vi "Get-Power.vi"(8 "error in":errorcluster, 11 "Average Time (0.0)":dbl=0.1) -> (0 "error out":errorcluster, 3 "Power":dbl)   [LabVIEW 2014]
uses:
  Global variables.vi
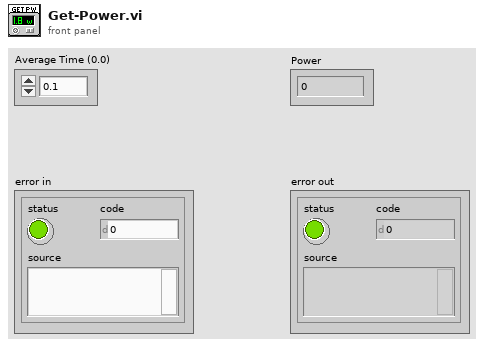
[diagram p1: front panel]
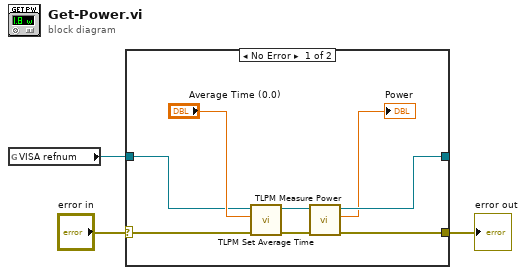
[diagram p0: block diagram]
diagram:
  n1 = global read "Global variables.vi" "VISA refnum"() -> (w1:refnum<visa-resource-name>)
  n2 = case shown="No Error" "error in" {
    selector: "error in" -> [w8 w12]
    tunnel: [w7 w12] -> w2
    tunnel: [w6 w13] -> _
    tunnel: w1 -> [w5 w13]
    frame No Error {
      n3 = call <instrlib>:"TLPM Set Average Time.vi"("error in (no error)"=w8, "Average Time (0.0)"="Average Time (0.0)", "instrument handle"=w5) -> ("error out"=w9:errorcluster, "instrument handle out"=w11:refnum<visa-resource-name>)  [unwired: 7 in]
      n4 = call "TLPM Measure Power.vi"("error in (no error)"=w9, "instrument handle"=w11) -> ("error out"=w7:errorcluster, "Power"=→"Power":dbl, "instrument handle out"=w6:refnum<visa-resource-name>)  [unwired: 7 in]
    }
    frame Error {
    }
  }
  "error out" <- w2
